vi "Read_BSA_setup.vi"(0 "GPIB Address":string, 5 "Multiply Velocity by -1":bool) -> (1 "Output":T1={"Output data format"=enum."Velocity", "Non-validated signals"=enum."Reject"}, 2 "Signal conditioning":T2={"High voltage"=2000, "Signal gain (dB)"=45} {"Signal gain (dB)" min=0 max=57 step=1; "High voltage" min=0 max=2040 step=8}, 3 "Anode current limit (mA)":T3(ring), 4 "Range":T7={"Centre Velocity"=16, "Velocity span"=10, "Units"=enum."m/s", "Frequency shift"=enum."Enabled"} {"Velocity span" items=["976.562E+0", "1.953E+3", "3.906E+3", "7.812E+3", "15.625E+3", "31.250E+3", "62.500E+3", "125.000E+3", "250.000E+3", "500.000E+3", "1.000E+6", "2.000E+6", "4.000E+6", "8.000E+6"]; "Centre Velocity" items=["0.000E+0", "0.000E+0", "0.000E+0", "0.000E+0", "0.000E+0", "0.000E+0", "0.000E+0", "0.000E+0", "0.000E+0", "0.000E+0", "0.000E+0", "0.000E+0"]}, 6 "Selected range":cluster{"Minimum":dbl, "Maximum":dbl}={"Minimum"=-1.9850000000000005, "Maximum"=1.9850000000000005} {"Maximum" format="%.2f"; "Minimum" format="%.2f"}, 8 "Clock parameters":T6={"Arrival time clock"=enum."Internal", "Clock source"=enum."Private", "Coincidence"=enum."Master"}, 9 "Centre frequency":dbl format="%.2f", 10 "Data collection mode":T5 {"Duty cycle (%)" format="%.2f"; "Dead time (s)" format="%.2f"}, 11 "Bandwidth":dbl format="%.2f", 12 "Setup string":string, 13 "Buffer mode":enum16{"One shot", "Ring", "FIFO"}(ring), 14 "Calibration factor":dbl=3.97 format="%.2f", 15 "Analysis parameters":T4={"Burst criterion"=enum."Envelope", "Oversize reject level"=enum."1 (disabled)", "Pedestal attenuation"=enum."0", "Record length"=enum."16", "Quality factor"=0} {"Quality factor" min=0 max=80 step=10})   [LabVIEW 2010]
panel:
  out "Read Info":string[][](array[string])
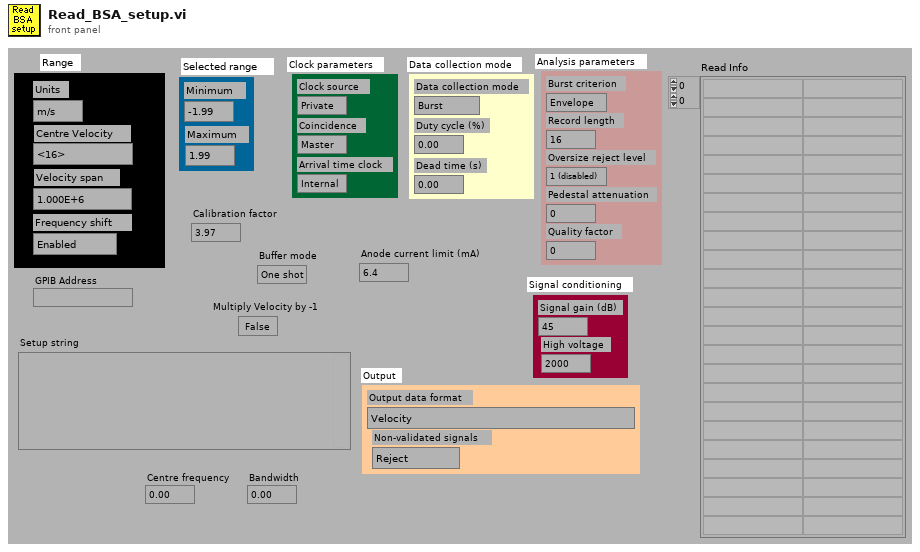
[diagram p1: front panel]
types:
  T1 = cluster{"Output data format":enum16{"Velocity, transit time, arrival time", "Velocity, arrival time", "Velocity, transit time", "Velocity"}, "Non-validated signals":enum16{"Accept", "Reject"}}
  T2 = cluster{"High voltage":i16, "Signal gain (dB)":i16}
  T3 = enum16{"6.4", "3.2", "1.6", "0.8", "0.4", "0.2", "0.1", "0.05"}
  T4 = cluster{"Burst criterion":enum16{"Envelope", "Pedestal", "Env and ped"}, "Oversize reject level":enum16{"1 (disabled)", "2", "3", "4", "5", "6", "7", "8", "9"}, "Pedestal attenuation":enum16{"0", "6", "12", "18"}, "Record length":enum16{"8", "16", "32", "64"}, "Quality factor":i16}
  T5 = cluster{"Dead time (s)":dbl, "Duty cycle (%)":dbl, "Data collection mode":enum16{"Burst", "Contiuous", "Dead time", "External"}}
  T6 = cluster{"Arrival time clock":enum16{"External", "Internal"}, "Clock source":enum16{"Slave", "Master", "Private"}, "Coincidence":enum16{"Slave", "Master", "Private"}}
  T7 = cluster{"Centre Velocity":u16, "Velocity span":u16, "Units":enum16{"Hz", "m/s"}, "Frequency shift":enum16{"Disabled", "Enabled"}}
  T8 = enum16{"CEN", "SPA", "SIG", "PED", "HIG", "REC", "MOD", "CAL", "WHO", "LOC", "REM"}
  T9 = cluster{"Centre frequency":u16, "Bandwidth":u16, "Units":enum16{"Hz", "m/s"}, "Frequency shift":enum16{"Disabled", "Enabled"}}
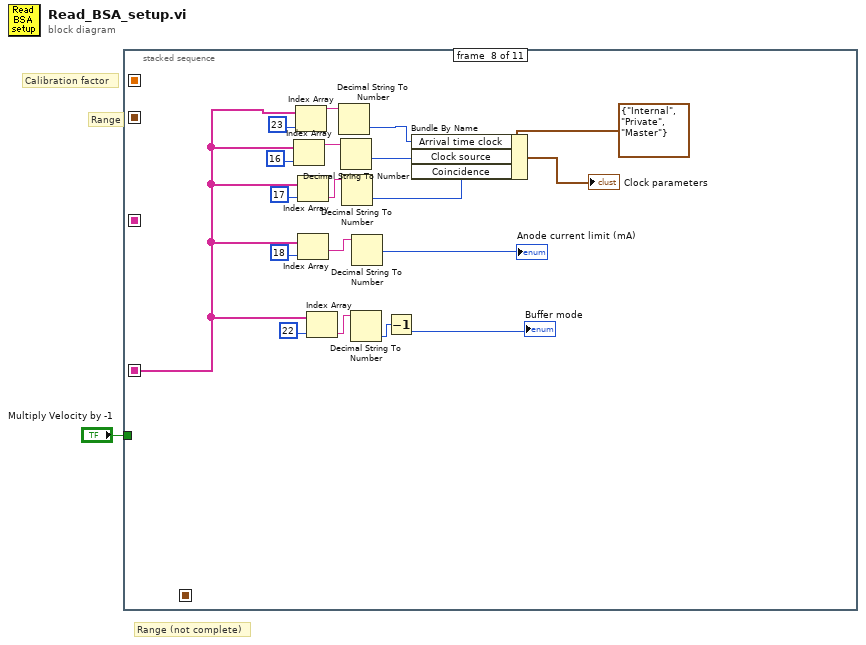
[diagram p0: block diagram]
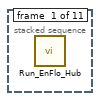
[diagram p2: hidden frame]
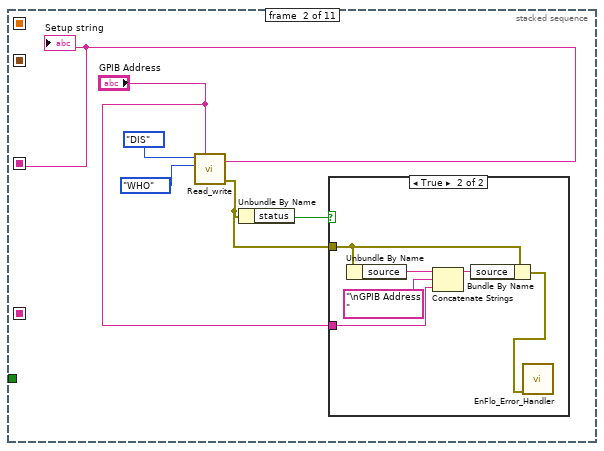
[diagram p3: hidden frame]
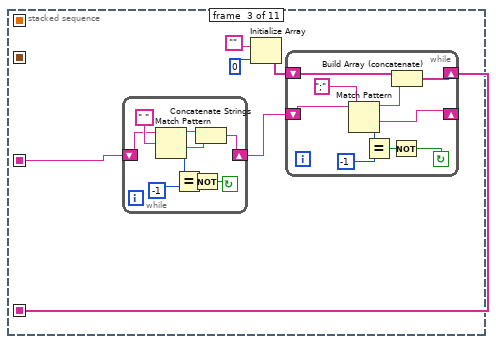
[diagram p5: hidden frame]
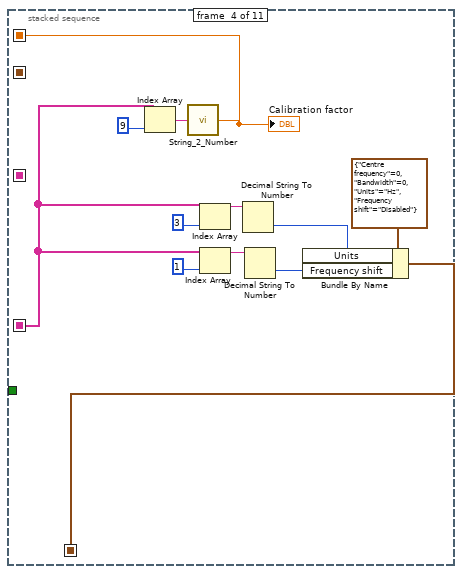
[diagram p6: hidden frame]
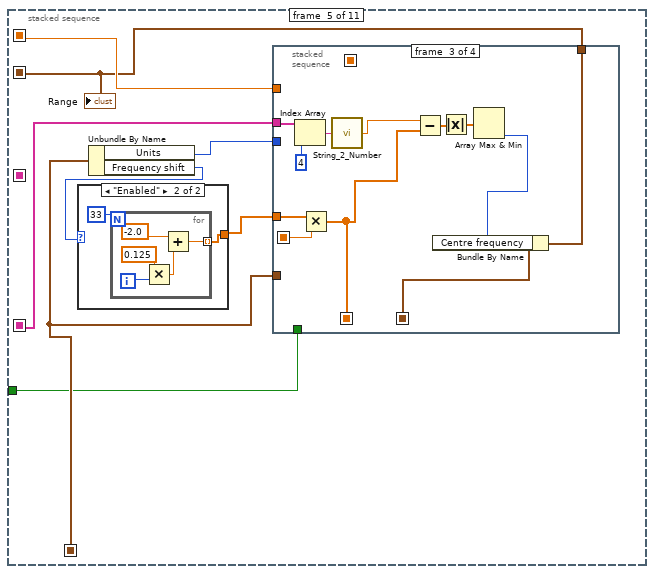
[diagram p7: hidden frame]
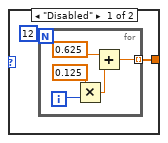
[diagram p8: hidden frame]
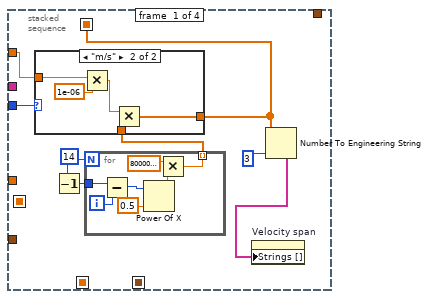
[diagram p9: hidden frame]
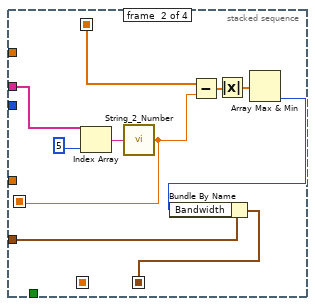
[diagram p11: hidden frame]
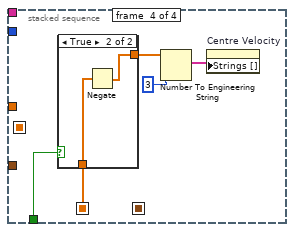
[diagram p12: hidden frame]
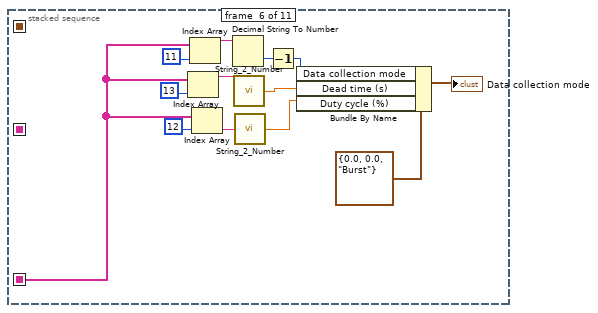
[diagram p14: hidden frame]
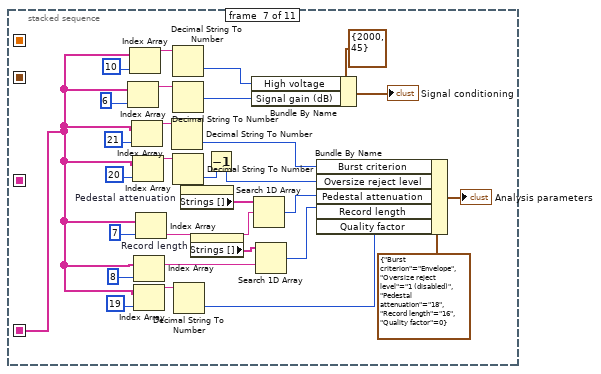
[diagram p15: hidden frame]
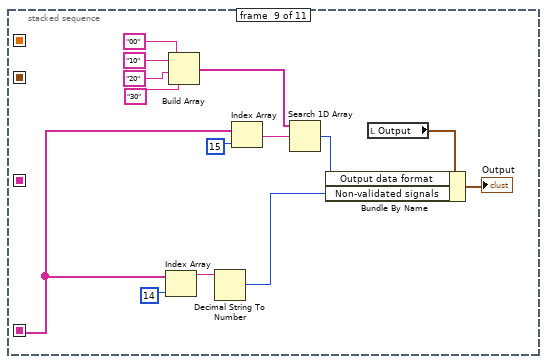
[diagram p16: hidden frame]
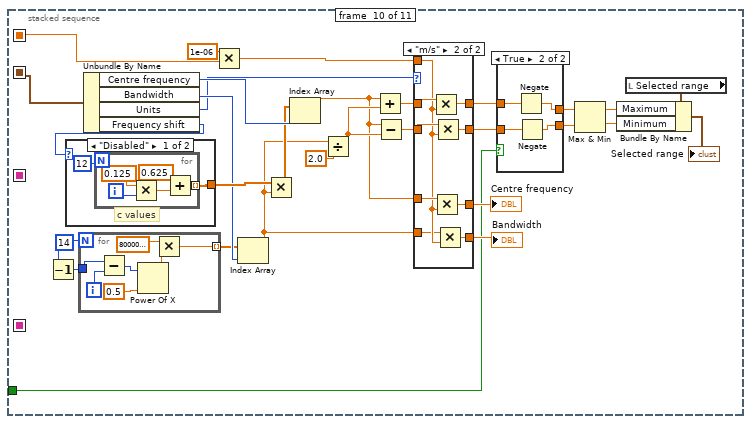
[diagram p17: hidden frame]
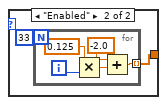
[diagram p20: hidden frame]
diagram:
  # "Range"
  # "Range (not complete)"
  # "Calibration factor"
  n1 = stacked-sequence {
    seq-local: [_ _ w16 _ _ _ _ _ _ _ _] -> [_ _ _ w42 w55 w124 w142 w167 w192 _ _]
    seq-local: [_ _ _ w39 _ _ _ _ _ _ _] -> [_ _ _ _ w56 _ _ _ _ w210 _]
    seq-local: [_ _ _ w40 _ _ _ _ _ _ _] -> [_ _ _ _ w54 _ _ _ _ _ _]
    seq-local: [_ _ _ _ w52 _ _ _ _ _ _] -> [_ _ _ _ _ _ _ _ _ w228 _]
    seq-local: [_ w7 _ _ _ _ _ _ _ _ _] -> [_ _ w14 _ _ _ _ _ _ _ w269]
    tunnel: "Multiply Velocity by -1" -> [_ _ _ _ w51 _ _ _ _ w205 _]
    frame #0 {
      n2 = call "Run_EnFlo_Hub.vi"() -> ()  [unwired: 8 out]
    }
    frame #1 {
      n3 = call "Read_write.vi"("Command"=enum16{"SET", "DIS"}."DIS", "Function"=T8."WHO", "GPIB address"="GPIB Address") -> ("Message received"=w7:string, "error out"=w3:errorcluster)  [unwired: 2 in]
      "Setup string" <- w7
      n4 = Unbundle By Name(w3) -> ("status"=w4:bool)
      n5 = case shown="True" w4 {
        tunnel: w3 -> [_ w13]
        tunnel: "GPIB Address" -> [_ w10]
        frame False {
        }
        frame True {
          n6 = Unbundle By Name(w13) -> ("source"=w12:string)
          n7 = Concatenate Strings(w12, "\nGPIB Address ", w10) -> (w9:string)
          n8 = Bundle By Name(cluster=w13, "source"=w9) -> (w8:errorcluster)
          n9 = call "EnFlo_Error_Handler.vi"("error in (no error)"=w8) -> ()  [unwired: 2 in, 3 out]
        }
      }
    }
    frame #2 {
      n10 = while {
        shift-left: w14 -> [w37]
        shift-right: [w34] -> w15
        stop <- w30 continue-if-true
        n11 = Match Pattern(string=w37, regular expression=" ") -> (before substring=w36:string, after substring=w35:string, offset past match=w33:i32)  [unwired: 2 out]
        n12 = Equal?(x=w33, y=-1) -> (x = y?=w31:bool)
        n13 = Not(x=w31) -> (.not. x?=w30:bool)
        n14 = Concatenate Strings(w36, w35) -> (w34:string)
      }
      n15 = Initialize Array("", 0) -> (w17:string[])
      n16 = while {
        shift-left: w17 -> [w28]
        shift-right: [w26] -> w16
        shift-left: w15 -> [w25]
        shift-right: [w29] -> _
        stop <- w20 continue-if-true
        n17 = Match Pattern(string=w25, regular expression=";") -> (before substring=w27:string, after substring=w29:string, offset past match=w22:i32)  [unwired: 2 out]
        n18 = Equal?(x=w22, y=-1) -> (x = y?=w21:bool)
        n19 = Not(x=w21) -> (.not. x?=w20:bool)
        n20 = Build Array (concatenate)(w28, w27) -> (w26:string[])
      }
    }
    frame #3 {
      n21 = Index Array(array=w42, index=9) -> (element=w49:string)
      n22 = call "String_2_Number.vi"("Value"=w49) -> ("Numeric"=w39:dbl)
      "Calibration factor" <- w39
      n23 = Index Array(array=w42, index=3) -> (element=w45:string)
      n24 = Index Array(array=w42, index=1) -> (element=w47:string)
      n25 = Decimal String To Number(string=w45) -> (number=w46:i32)  [unwired: 3 out]
      n26 = Decimal String To Number(string=w47) -> (number=w48:i32)  [unwired: 3 out]
      n27 = Bundle By Name(cluster=T9 {"Centre frequency"=0, "Bandwidth"=0, "Units"=enum."Hz", "Frequency shift"=enum."Disabled"} ("Range"), "Units"=w46, "Frequency shift"=w48) -> (w40:T9)
    }
    frame #4 {
      n28 = Unbundle By Name(w54) -> ("Units"=w57:enum16{"Hz", "m/s"}, "Frequency shift"=w58:enum16{"Disabled", "Enabled"})
      n29 = case shown="\"Enabled\"" w58 {
        tunnel: [w59 w66] -> w53
        frame "Disabled" {
          n30 = for {
            N: 12 -> [_]
            tunnel: [w61] -> w59 mode=indexing
            i -> [w62]
            n31 = Multiply(x=0.125, y=w62) -> (x*y=w64:dbl)
            n32 = Add(x=0.625, y=w64) -> (x+y=w61:dbl)
          }
        }
        frame "Enabled" {
          n33 = for {
            N: 33 -> [_]
            tunnel: [w68] -> w66 mode=indexing
            i -> [w69]
            n34 = Multiply(x=0.125, y=w69) -> (x*y=w71:dbl)
            n35 = Add(x=-2.0, y=w71) -> (x+y=w68:dbl)
          }
        }
      }
      n36 = stacked-sequence {
        seq-local: [_ w96 _ _] -> [_ _ w114 _]
        seq-local: [w74 _ _ _] -> [_ w94 _ _]
        seq-local: [_ w99 _ _] -> [_ _ w106 _]
        seq-local: [_ _ w104 _] -> [_ _ _ w117]
        tunnel: w56 -> [w80 _ _ _]
        tunnel: w57 -> [w75 _ _ _]
        tunnel: w55 -> [_ w101 w111 _]
        tunnel: w53 -> [_ _ w115 _]
        tunnel: w54 -> [_ w100 _ _]
        tunnel: [_ _ w105 _] -> w52
        tunnel: w51 -> [_ _ _ w118]
        frame #0 {
          w76 = 14
          n37 = Decrement(x=w76) -> (x-1=w77:i32)
          n38 = for {
            N: w76 -> [_]
            tunnel: w77 -> [w88]
            tunnel: [w87] -> w78 mode=indexing
            i -> [w93]
            n39 = Subtract(x=w88, y=w93) -> (x-y=w91:i32)
            n40 = Power Of X(1:0.5, 2:w91) -> (0:w90:dbl)
            n41 = Multiply(x=8000000.0, y=w90) -> (x*y=w87:dbl)
          }
          n42 = case shown="\"m/s\"" w75 {
            tunnel: w78 -> [w81 w86]
            tunnel: [w81 w83] -> w74
            tunnel: w80 -> [_ w82]
            frame "Hz" {
            }
            frame "m/s" {
              n43 = Multiply(x=w82, y=1e-06) -> (x*y=w84:dbl)
              n44 = Multiply(x=w84, y=w86) -> (x*y=w83:dbl[])
            }
          }
          n45 = Number To Engineering String(2:3, 4:w74) -> (0:w73:string[])  [unwired: 2 out]
          n46 = property on="Velocity span" class="Ring (strict)"("Strings []"=w73) -> ()  [unwired: 2 in, 2 out]
        }
        frame #1 {
          n47 = Index Array(array=w101, index=5) -> (element=w102:string)
          n48 = call "String_2_Number.vi"("Value"=w102) -> ("Numeric"=w96:dbl)
          n49 = Subtract(x=w94, y=w96) -> (x-y=w98:dbl[])
          n50 = Absolute Value(x=w98) -> (abs(x)=w97:dbl[])
          n51 = Array Max & Min(array=w97) -> (min index (indices)=w95:i32)  [unwired: 3 out]
          n52 = Bundle By Name(cluster=w100, "Bandwidth"=w95) -> (w99:T9)
        }
        frame #2 {
          n53 = Index Array(array=w111, index=4) -> (element=w112:string)
          n54 = Multiply(x=w115, y=w114) -> (x*y=w104:dbl[])
          n55 = call "String_2_Number.vi"("Value"=w112) -> ("Numeric"=w110:dbl)
          n56 = Subtract(x=w110, y=w104) -> (x-y=w109:dbl[])
          n57 = Absolute Value(x=w109) -> (abs(x)=w108:dbl[])
          n58 = Array Max & Min(array=w108) -> (min index (indices)=w107:i32)  [unwired: 3 out]
          n59 = Bundle By Name(cluster=w106, "Centre frequency"=w107) -> (w105:T9)
        }
        frame #3 {
          n60 = case shown="True" w118 {
            tunnel: w117 -> [w121 w123]
            tunnel: [w121 w122] -> w116
            frame False {
            }
            frame True {
              n61 = Negate(x=w123) -> (-x=w122:dbl[])
            }
          }
          n62 = Number To Engineering String(2:3, 4:w116) -> (0:w119:string[])  [unwired: 2 out]
          n63 = property on="Centre Velocity" class="Ring (strict)"("Strings []"=w119) -> ()  [unwired: 2 in, 2 out]
        }
      }
      "Range" <- w52
    }
    frame #5 {
      n64 = Index Array(array=w124, index=13) -> (element=w129:string)
      n65 = Index Array(array=w124, index=11) -> (element=w127:string)
      n66 = Index Array(array=w124, index=12) -> (element=w131:string)
      n67 = Decimal String To Number(string=w127) -> (number=w133:i32)  [unwired: 3 out]
      n68 = call "String_2_Number.vi"("Value"=w129) -> ("Numeric"=w130:dbl)
      n69 = call "String_2_Number.vi"("Value"=w131) -> ("Numeric"=w132:dbl)
      n70 = Decrement(x=w133) -> (x-1=w134:i32)
      n71 = Bundle By Name(cluster=T5 {"Dead time (s)"=0.0, "Duty cycle (%)"=0.0, "Data collection mode"=enum."Burst"} ("Data collection mode"), "Data collection mode"=w134, "Dead time (s)"=w130, "Duty cycle (%)"=w132) -> (→"Data collection mode":T5)
    }
    frame #6 {
      n72 = Index Array(array=w142, index=6) -> (element=w146:string)
      n73 = Index Array(array=w142, index=10) -> (element=w145:string)
      n74 = Index Array(array=w142, index=21) -> (element=w148:string)
      n75 = Index Array(array=w142, index=20) -> (element=w152:string)
      n76 = Index Array(array=w142, index=8) -> (element=w164:string)
      n77 = Index Array(array=w142, index=19) -> (element=w153:string)
      n78 = Index Array(array=w142, index=7) -> (element=w162:string)
      n79 = Decimal String To Number(string=w148) -> (number=w154:i32)  [unwired: 3 out]
      n80 = Decimal String To Number(string=w145) -> (number=w149:i32)  [unwired: 3 out]
      n81 = Decimal String To Number(string=w146) -> (number=w150:i32)  [unwired: 3 out]
      n82 = Decimal String To Number(string=w152) -> (number=w155:i32)  [unwired: 3 out]
      n83 = Decimal String To Number(string=w153) -> (number=w157:i32)  [unwired: 3 out]
      n84 = property on="Pedestal attenuation" class="Enum (strict)"() -> ("Strings []"=w141:string[])  [unwired: 2 in, 2 out]
      n85 = property on="Record length" class="Enum (strict)"() -> ("Strings []"=w140:string[])  [unwired: 2 in, 2 out]
      n86 = Decrement(x=w155) -> (x-1=w156:i32)
      n87 = Bundle By Name(cluster=T2 {"High voltage"=2000, "Signal gain (dB)"=45} ("Signal conditioning"), "High voltage"=w149, "Signal gain (dB)"=w150) -> (→"Signal conditioning":T2)
      n88 = Search 1D Array(1D array=w141, element=w162) -> (index of element=w163:i32)  [unwired: 1 out]
      n89 = Search 1D Array(1D array=w140, element=w164) -> (index of element=w165:i32)  [unwired: 1 out]
      n90 = Bundle By Name(cluster=T4 {"Burst criterion"=enum."Envelope", "Oversize reject level"=enum."1 (disabled)", "Pedestal attenuation"=enum."18", "Record length"=enum."16", "Quality factor"=0} ("Analysis parameters"), "Burst criterion"=w154, "Oversize reject level"=w156, "Pedestal attenuation"=w163, "Record length"=w165, "Quality factor"=w157) -> (→"Analysis parameters":T4)
    }
    frame #7 {
      n91 = Index Array(array=w167, index=16) -> (element=w173:string)
      n92 = Index Array(array=w167, index=23) -> (element=w170:string)
      n93 = Index Array(array=w167, index=17) -> (element=w174:string)
      n94 = Index Array(array=w167, index=18) -> (element=w181:string)
      n95 = Index Array(array=w167, index=22) -> (element=w178:string)
      n96 = Decimal String To Number(string=w170) -> (number=w171:i32)  [unwired: 3 out]
      n97 = Decimal String To Number(string=w173) -> (number=w175:i32)  [unwired: 3 out]
      n98 = Decimal String To Number(string=w174) -> (number=w176:i32)  [unwired: 3 out]
      n99 = Decimal String To Number(string=w178) -> (number=w180:i32)  [unwired: 3 out]
      n100 = Decimal String To Number(string=w181) -> (number=→"Anode current limit (mA)":i32)  [unwired: 3 out]
      n101 = Decrement(x=w180) -> (x-1=→"Buffer mode":i32)
      n102 = Bundle By Name(cluster=T6 {"Arrival time clock"=enum."Internal", "Clock source"=enum."Private", "Coincidence"=enum."Master"} ("Clock parameters"), "Arrival time clock"=w171, "Clock source"=w175, "Coincidence"=w176) -> (→"Clock parameters":T6)
    }
    frame #8 {
      n103 = Index Array(array=w192, index=14) -> (element=w191:string)
      n104 = Build Array("00", "10", "20", "30") -> (w189:string[])
      n105 = Decimal String To Number(string=w191) -> (number=w186:i32)  [unwired: 3 out]
      n106 = Index Array(array=w192, index=15) -> (element=w188:string)
      n107 = Search 1D Array(1D array=w189, element=w188) -> (index of element=w187:i32)  [unwired: 1 out]
      n108 = local read "Output"() -> (w190:T1)
      n109 = Bundle By Name(cluster=w190, "Output data format"=w187, "Non-validated signals"=w186) -> (→"Output":T1)
    }
    frame #9 {
      w218 = 14
      n110 = Decrement(x=w218) -> (x-1=w219:i32)
      n111 = for {
        N: w218 -> [_]
        tunnel: w219 -> [w249]
        tunnel: [w248] -> w213 mode=indexing
        i -> [w254]
        n112 = Subtract(x=w249, y=w254) -> (x-y=w252:i32)
        n113 = Power Of X(1:0.5, 2:w252) -> (0:w251:dbl)
        n114 = Multiply(x=8000000.0, y=w251) -> (x*y=w248:dbl)
      }
      n115 = Unbundle By Name(w228) -> ("Centre frequency"=w226:u16, "Bandwidth"=w225:u16, "Units"=w214:enum16{"Hz", "m/s"}, "Frequency shift"=w224:enum16{"Disabled", "Enabled"})
      n116 = case shown="\"Disabled\"" w224 {
        tunnel: [w255 w262] -> w227
        frame "Disabled" {
          # "c values"
          n117 = for {
            N: 12 -> [_]
            tunnel: [w257] -> w255 mode=indexing
            i -> [w258]
            n118 = Multiply(x=0.125, y=w258) -> (x*y=w260:dbl)
            n119 = Add(x=0.625, y=w260) -> (x+y=w257:dbl)
          }
        }
        frame "Enabled" {
          n120 = for {
            N: 33 -> [_]
            tunnel: [w264] -> w262 mode=indexing
            i -> [w265]
            n121 = Multiply(x=0.125, y=w265) -> (x*y=w267:dbl)
            n122 = Add(x=-2.0, y=w267) -> (x+y=w264:dbl)
          }
        }
      }
      n123 = Multiply(x=1e-06, y=w210) -> (x*y=w212:dbl)
      n124 = Index Array(array=w213, index=w225) -> (element=w208:dbl)
      n125 = Multiply(x=w227, y=w208) -> (x*y=w211:dbl[])
      n126 = Index Array(array=w211, index=w226) -> (element=w209:dbl)
      n127 = Divide(x=w208, y=2.0) -> (x/y=w221:dbl)
      n128 = Add(x=w209, y=w221) -> (x+y=w216:dbl)
      n129 = Subtract(x=w209, y=w221) -> (x-y=w215:dbl)
      n130 = case shown="\"m/s\"" w214 {
        tunnel: w216 -> [w238 w247]
        tunnel: w215 -> [w237 w246]
        tunnel: [w238 w245] -> w203
        tunnel: [w237 w244] -> w204
        tunnel: w212 -> [_ w242]
        tunnel: w209 -> [w236 w243]
        tunnel: w208 -> [w235 w241]
        tunnel: [w235 w240] -> w207
        tunnel: [w236 w239] -> w206
        frame "Hz" {
        }
        frame "m/s" {
          n131 = Multiply(x=w247, y=w242) -> (x*y=w245:dbl)
          n132 = Multiply(x=w243, y=w242) -> (x*y=w239:dbl)
          n133 = Multiply(x=w246, y=w242) -> (x*y=w244:dbl)
          n134 = Multiply(x=w241, y=w242) -> (x*y=w240:dbl)
        }
      }
      "Centre frequency" <- w206
      "Bandwidth" <- w207
      n135 = case shown="True" w205 {
        tunnel: w204 -> [w229 w234]
        tunnel: w203 -> [w230 w233]
        tunnel: [w230 w232] -> w202
        tunnel: [w229 w231] -> w201
        frame False {
        }
        frame True {
          n136 = Negate(x=w233) -> (-x=w232:dbl)
          n137 = Negate(x=w234) -> (-x=w231:dbl)
        }
      }
      n138 = Max & Min(x=w202, y=w201) -> (max(x,y)=w200:dbl, min(x,y)=w199:dbl)
      n139 = local read "Selected range"() -> (w223:cluster{"Minimum":dbl, "Maximum":dbl})
      n140 = Bundle By Name(cluster=w223, "Maximum"=w200, "Minimum"=w199) -> (→"Selected range":cluster{"Minimum":dbl, "Maximum":dbl})
    }
    frame #10 {
      n141 = for {
        shift-right: [w276] -> _
        shift-left: w269 -> [w277]
        tunnel: string[][] [["0", "BSA"], ["1", "Frequency shift"], ["2", "IEEE time delay"], ["3", "Units"], ["4", "Velocity Centre"], ["5", "Velocity Span"], ["6", "Signal Gain"], ["7", "Pedestal Attenuation"], ["8", "Record Length"], ["9", "Calibration factor"], ["10", "High Voltage"], ["11", "Data collection mode"], ["12", "Duty cycle (%)"], ["13", "Dead time (s)"], ["14", "Non-validation signals"], ["15", "Output data format"], ["16", "Clock source"], ["17", "Coincidence"], ["18", "Anode current limit"], ["19", "Quality Factor"], ["20", "Oversize rejection"], ["21", "Burst Criterion"], ["22", "Buffer mode"], ["23", "Arrival time clock"]] -> [w275] mode=indexing
        tunnel: [w273] -> w271 mode=indexing
        n142 = Match Pattern(string=w277, regular expression=";") -> (before substring=w274:string, after substring=w276:string)  [unwired: 3 out]
        n143 = Build Array (concatenate)(w275, w274) -> (w273:string[])
      }
      "Read Info" <- w271
    }
  }
